vi "Galil event_onMessage.vi"(4 "message":refnum<vi>, 5 "Event Data":cluster{"message":string}, 6 "Control Ref":refnum<k7>, 7 "Event Common Data":T1) -> ()   [LabVIEW 2011]
panel:
  out "error out":errorcluster
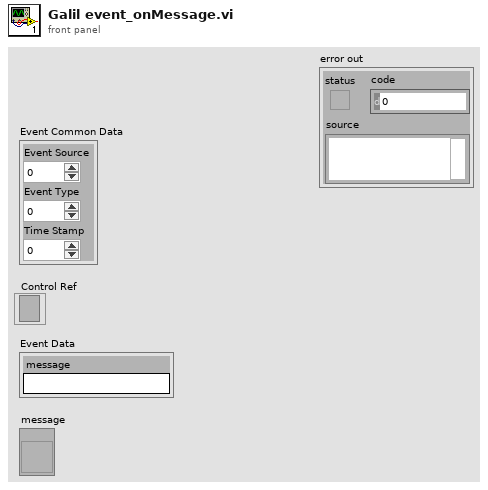
[diagram p1: front panel]
types:
  T1 = cluster{"Event Source":i32, "Event Type":u32, "Time Stamp":u32}
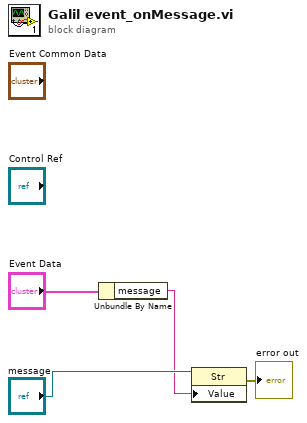
[diagram p0: block diagram]
diagram:
  n1 = Unbundle By Name("Event Data") -> ("message"=w2:string)
  n2 = property class="Str"(reference="message", "Value"=w2) -> (error out=→"error out":errorcluster)  [unwired: 1 in, 1 out]
